vi "Store Error - INI.vi"(4 "error in (no error)":errorcluster) -> (0 "error out":errorcluster)   [LabVIEW 2015, in "Error Reporting and Storage.lvlib"]
uses:
  Error Reporting and Storage.lvlib
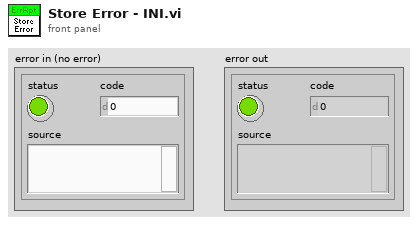
[diagram p1: front panel]
types:
  T1 = enum16{"open", "replace", "create", "open or create", "replace or create", "replace or create with confirmation"}
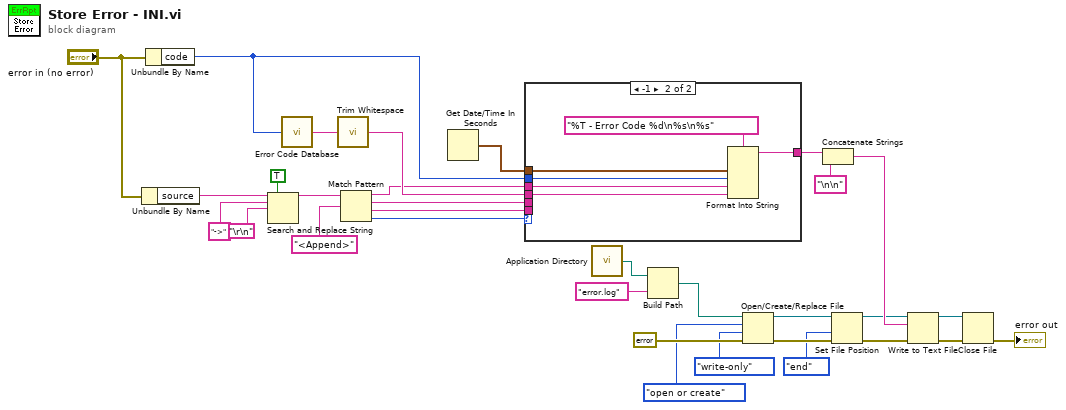
[diagram p0: block diagram]
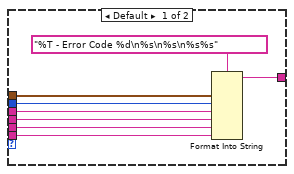
[diagram p2: hidden frame]
diagram:
  n1 = Unbundle By Name("error in (no error)") -> ("source"=w21:string)
  n2 = Unbundle By Name("error in (no error)") -> ("code"=w19:i32)
  n3 = Search and Replace String(replace all?=TRUE ("replace all? (F)"), input string=w21, search string="->", replace string="\r\n") -> (result string=w20:string)  [unwired: 4 in, 3 out]
  n4 = call <vilib>:"Error Code Database.vi"("Error Code"=w19) -> ("Error Text"=w32:string)
  n5 = call <vilib>:"Trim Whitespace.vi"("string"=w32) -> ("trimmed string"=w28:string)  [unwired: 1 in]
  n6 = Match Pattern(string=w20, regular expression="<Append>") -> (before substring=w25:string, match substring=w27:string, after substring=w26:string, offset past match=w30:i32)  [unwired: 1 in]
  n7 = Get Date/Time In Seconds() -> (seconds since 1Jan1904=w1:timestamp)
  n8 = case shown="-1" w30 {
    tunnel: w28 -> [w39 w44]
    tunnel: [w36 w45] -> w9
    tunnel: w27 -> [w38 _]
    tunnel: w26 -> [w37 _]
    tunnel: w25 -> [w35 w43]
    tunnel: w19 -> [w34 w42]
    tunnel: w1 -> [w33 w41]
    frame Default {
      n9 = Format Into String(format string="%T - Error Code %d\n%s\n%s\n%s%s", w33, w34, w35, w39, w38, w37) -> (resulting string=w36:string)  [unwired: 2 in, 1 out]
    }
    frame -1 {
      n10 = Format Into String(format string="%T - Error Code %d\n%s\n%s", w41, w42, w43, w44) -> (resulting string=w45:string)  [unwired: 2 in, 1 out]
    }
  }
  n11 = call <vilib>:"Application Directory.vi"() -> ("Application Directory"=w18:path)
  n12 = Build Path(base path=w18, name or relative path="error.log") -> (appended path=w16:path)
  n13 = Open/Create/Replace File(file path (use dialog)=w16, error in=errorcluster {"status"=FALSE, "code"=0, "source"=""} ("error constant"), operation (0:open)=T1."open or create", access (0:read/write)=enum16{"read/write", "read-only", "write-only"}."write-only") -> (refnum out=w5:refnum<file>, error out=w6:errorcluster)  [unwired: 2 in, 1 out]
  n14 = Concatenate Strings(w9, "\n\n" ("string")) -> (w7:string)
  n15 = Set File Position(refnum=w5, from (0:start)=enum16{"start", "end", "current"}."end", error in=w6) -> (refnum out=w4:refnum<file>, error out=w3:errorcluster)  [unwired: 1 in]
  n16 = Write to Text File(file (use dialog)=w4, text=w7, error in=w3) -> (refnum out=w10:refnum<file>, error out=w11:errorcluster)  [unwired: 1 in, 1 out]
  n17 = Close File(refnum=w10, error in=w11) -> (error out=→"error out":errorcluster)  [unwired: 1 out]
